vi "RT Comm Loop.vi"(11 "Queue in":refnum<queue>) -> ()   [LabVIEW 2014]
uses:
  Controls/RT Comm States.ctl
  Controls/RT Stream Data.ctl
  RT Stop.vi
  RT Comm Refs.vi
  <resource>/objmgr/ni.dex.rc
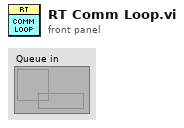
[diagram p1: front panel]
types:
  T1 = typedef "RT Comm States.ctl" = enum16{"Init", "Handshake", "Transfer"}
  T2 = typedef "RT Stream Data.ctl" = cluster{"Temp Data":dbl[], "pH Data":dbl[]}
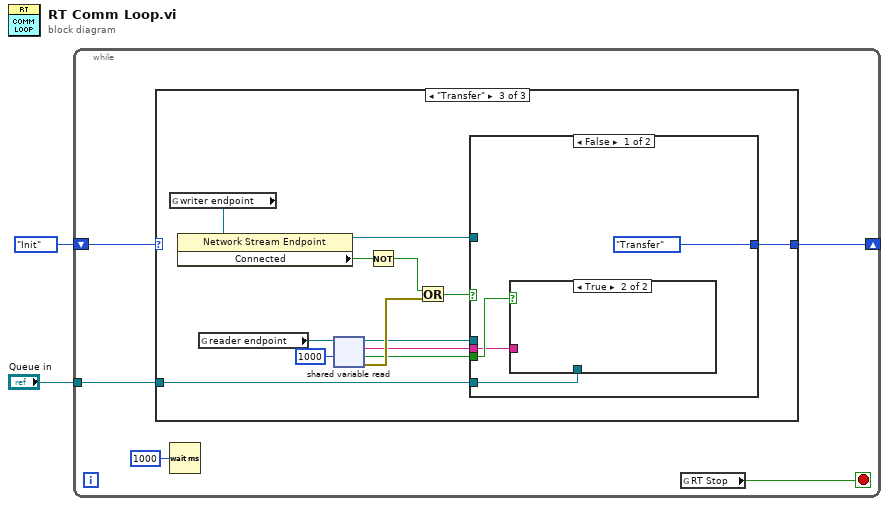
[diagram p0: block diagram]
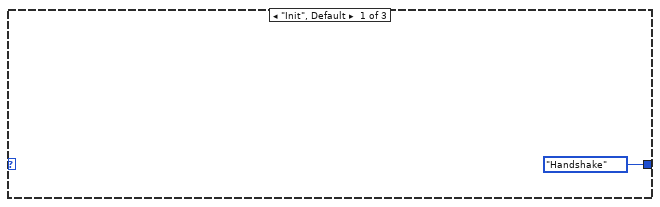
[diagram p2: hidden frame]
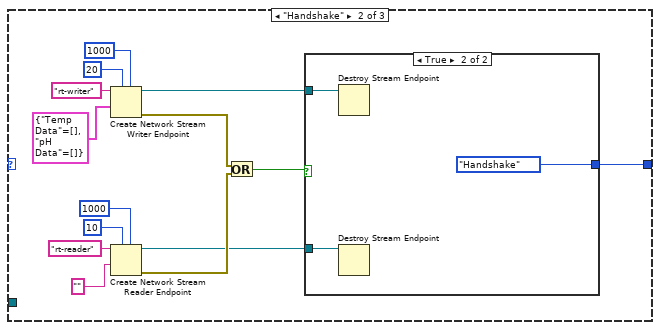
[diagram p3: hidden frame]
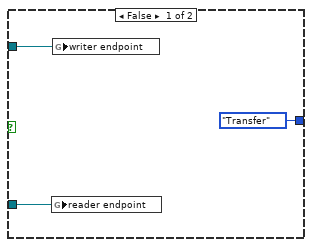
[diagram p4: hidden frame]
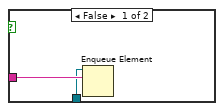
[diagram p5: hidden frame]
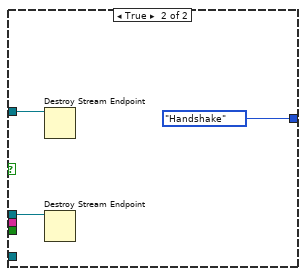
[diagram p6: hidden frame]
diagram:
  n1 = while {
    shift-right: [w5] -> _
    shift-left: RT_Comm_States."Init" -> [w7]
    tunnel: "Queue in" -> [w3]
    stop <- w6 stop-if-true
    n2 = case shown="\"Transfer\"" w7 {
      tunnel: [RT_Comm_States."Handshake" w9 w33] -> w5
      tunnel: w3 -> [_ _ w29]
      frame "Init", Default {
      }
      frame "Handshake" {
        n3 = Create Network Stream Writer Endpoint(5:1000 ("timeout in ms (-1)"), 7:20 ("writer buffer size"), 9:T2 {"Temp Data"=[], "pH Data"=[]} ("cluster"), 11:"rt-writer" ("writer name")) -> (0:w14:errorcluster, 3:w11:refnum<k21>)  [unwired: 3 in]
        n4 = Create Network Stream Reader Endpoint(5:1000 ("timeout in ms (-1)"), 7:10 ("reader buffer size"), 9:"", 11:"rt-reader" ("reader name")) -> (0:w13:errorcluster, 3:w10:refnum<k21>)  [unwired: 3 in]
        n5 = Or(x=w14, y=w13) -> (x .or. y?=w12:bool)
        n6 = case shown="True" w12 {
          tunnel: w11 -> [w25 w28]
          tunnel: w10 -> [w24 w27]
          tunnel: [RT_Comm_States."Transfer" RT_Comm_States."Handshake"] -> w9
          frame False {
            n7 = global write "RT Comm Refs.vi" "reader endpoint"(w24) -> ()
            n8 = global write "RT Comm Refs.vi" "writer endpoint"(w25) -> ()
          }
          frame True {
            n9 = Destroy Stream Endpoint(11:w28) -> ()  [unwired: 1 in, 1 out]
            n10 = Destroy Stream Endpoint(11:w27) -> ()  [unwired: 1 in, 1 out]
          }
        }
      }
      frame "Transfer" {
        n11 = global read "RT Comm Refs.vi" "writer endpoint"() -> (w39:refnum<k21>)
        n12 = property class="Network Stream Endpoint"(reference=w39) -> (reference out=w34:refnum<k21>, "Connected"=w38:bool)  [unwired: 1 in, 1 out]
        n13 = global read "RT Comm Refs.vi" "reader endpoint"() -> (w41:refnum<k21>)
        n14 = shared-variable-read(w41, 1000 ("timeout ms (-1)")) -> (w32:refnum<k21>, w36:errorcluster, w30:bool, w31:string)  [unwired: 1 in]
        n15 = Not(x=w38) -> (.not. x?=w37:bool)
        n16 = Or(x=w37, y=w36) -> (x .or. y?=w35:bool)
        n17 = case shown="False" w35 {
          tunnel: w34 -> [_ w50]
          tunnel: [RT_Comm_States."Transfer" RT_Comm_States."Handshake"] -> w33
          tunnel: w32 -> [_ w48]
          tunnel: w31 -> [w43 _]
          tunnel: w30 -> [w45 _]
          tunnel: w29 -> [w42 _]
          frame False {
            n18 = case shown="True" w45 {
              tunnel: w43 -> [w47 _]
              tunnel: w42 -> [w46 _]
              frame False {
                n19 = Enqueue Element(queue=w46, element=w47) -> ()  [unwired: 2 in, 3 out]
              }
              frame True {
              }
            }
          }
          frame True {
            n20 = Destroy Stream Endpoint(11:w50) -> ()  [unwired: 1 in, 1 out]
            n21 = Destroy Stream Endpoint(11:w48) -> ()  [unwired: 1 in, 1 out]
          }
        }
      }
    }
    n22 = Wait (ms)(milliseconds to wait=u32 1000) -> ()  [unwired: 1 out]
    n23 = global read "RT Stop.vi" "RT Stop"() -> (w6:bool)
  }
